vi "PUBLIC.constructor.vi"(0 "name":string, 2 "data in":string, 5 "error in(no error)":errorcluster) -> (14 "i ref out":refnum<vi>, 16 "data out":string, 19 "error out":errorcluster)   [LabVIEW 2014, in "PTScanner.lvlib"]
doc: "This is the constructor of a class.\n\nLicense Agreement for this software:\n\nCopyright (C)\nGesellschaft für Schwerionenforschung, GSI\nPlanckstr. 1\n64291 Darmstadt\nGermany\n\nContact: D.Beck@gsi.de \n\nThis program is free software; you can redistribute it and/or modify it under the terms of the \nGNU General Public License as published by the Free Software Foundation; either version 2 of \nthe license, or (at your option) any later version.\n\nThis program is distributed in the hope that it will be useful, but WITHOUT ANY WARRANTY; \nwithout even the implied warranty of MERCHANTABILITY or FITNESS FOR A PARTICULAR PURPOSE. See the GNU General License for more details (http://www.gnu.org).\n\nGesellschaft für Schwerionenforschung, GSI\nPlanckstr. 1, 64291 Darmstadt, Germany\nFor all questions and ideas contact: M.Richter@gsi.de, H.Brand@gsi.de or D.Beck@gsi.de.\nLast update: 16-JUN-2004"
uses:
  PTScanner.lvlib
  CS_Core/CSSystem/CSSystemLib/CSSystemLib.lvlib
  CS_Core/BaseProcess/BaseProcess.lvlib
  CS_Core/CSObj/CSObj.lvlib
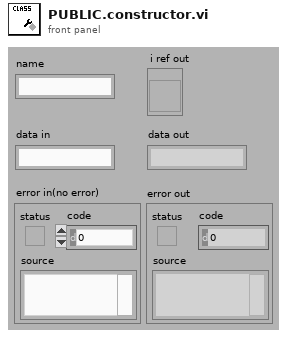
[diagram p1: front panel]
types:
  T1 = enum16{"SetAttribute", "GetAttribute", "CreateAttribute", "DestroyAttribute", "DestroyAllAtributes"}
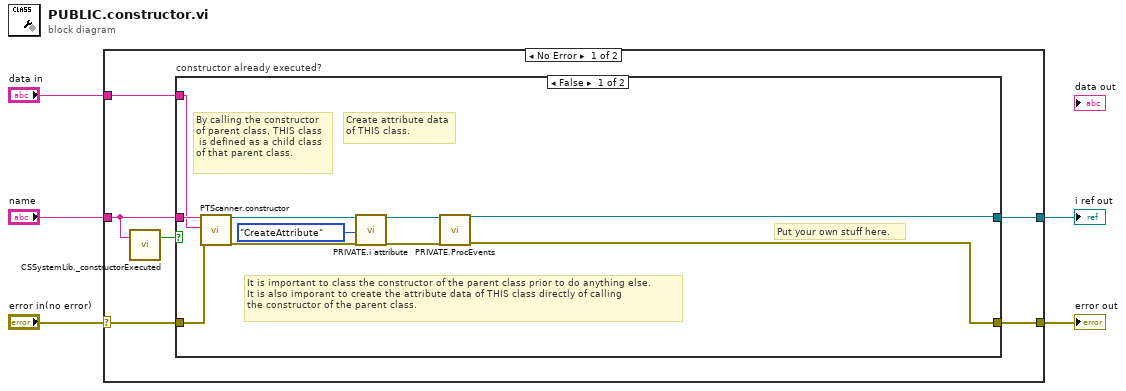
[diagram p0: block diagram]
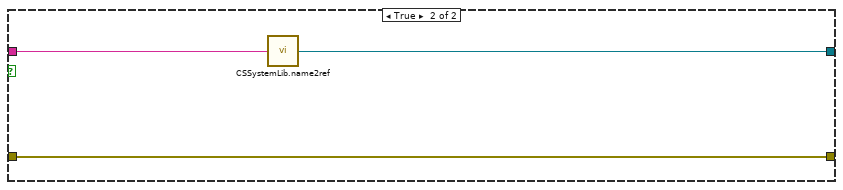
[diagram p2: hidden frame]
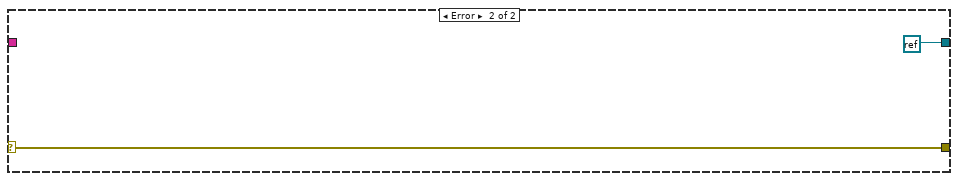
[diagram p3: hidden frame]
diagram:
  n1 = case shown="No Error" "error in(no error)" {
    selector: "error in(no error)" -> [w9 w25]
    tunnel: "name" -> [w8 _]
    tunnel: [w11 refnum<k0> refnum] -> w4
    tunnel: [w10 w25] -> w3
    tunnel: "data in" -> [w6 _]
    frame No Error {
      n2 = call "CSSystemLib._constructorExecuted.vi"("name"=w8) -> ("constructor executed?"=w7:bool)  [unwired: 18 in]
      n3 = case "constructor already executed?" shown="False" w7 {
        tunnel: w8 -> [w21 w24]
        tunnel: [w13 w23] -> w11
        tunnel: [w12 w22] -> w10
        tunnel: w9 -> [w20 w22]
        tunnel: w6 -> [w19 _]
        frame False {
          # "It is important to class the constructor of the parent class prior to do anything else.\nIt is also imporant to create the attribute data of THIS class directly of calling\nthe constructor of the parent class."
          # "Put your own stuff here."
          # "Create attribute data\nof THIS class."
          # "By calling the constructor\nof parent class, THIS class\n is defined as a child class\nof that parent class."
          n4 = call "PTScanner.constructor.vi"("name"=w21, "data in"=w19, "error in(no error)"=w20) -> ("i ref out"=w16:refnum<vi>, "error out"=w18:errorcluster)  [unwired: 14 in, 1 out]
          n5 = call "PRIVATE.i attribute.vi"("VI Refnum"=w16, "Action"=T1."CreateAttribute", "error in (no error)"=w18) -> ("VI Refnum out"=w15:refnum<vi>, "error out"=w14:errorcluster)  [unwired: 14 in, 1 out]
          n6 = call "PRIVATE.ProcEvents.vi"("i ref in"=w15, "error in (no error)"=w14) -> ("i ref out"=w13:refnum<vi>, "error out"=w12:errorcluster)  [unwired: 16 in]
        }
        frame True {
          n7 = call "CSSystemLib.name2ref.vi"("name"=w24) -> ("obj refnum"=w23:refnum<vi>)
        }
      }
    }
    frame Error {
    }
  }
  "i ref out" <- w4
  "error out" <- w3
